vi "Build keyword and value string vector.vi"(1 "Keywords":string, 3 "Values":string) -> (15 "Keywords & Values in 128 Bytes vector":u8[](array[numeric]))   [LabVIEW 2022 SP3, in "RPC.lvclass"]
uses:
  RPC.lvclass
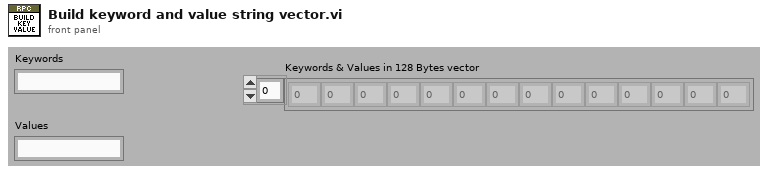
[diagram p1: front panel]
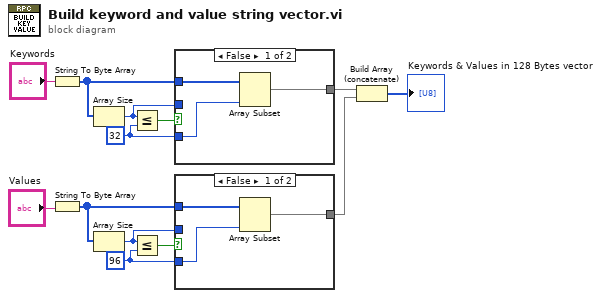
[diagram p0: block diagram]
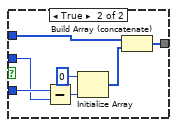
[diagram p2: hidden frame]
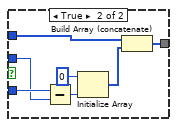
[diagram p3: hidden frame]
diagram:
  w7 = 96 ("y")
  w10 = 32 ("y")
  n1 = String To Byte Array(string="Keywords") -> (unsigned byte array=w11:u8[])
  n2 = String To Byte Array(string="Values") -> (unsigned byte array=w6:u8[])
  n3 = Array Size(array=w11) -> (size(s)=w9:i32)
  n4 = Array Size(array=w6) -> (size(s)=w8:i32)
  n5 = Less Or Equal?(x=w9, y=w10) -> (x <= y?=w12:bool)
  n6 = Less Or Equal?(x=w8, y=w7) -> (x <= y?=w5:bool)
  n7 = case shown="False" w12 {
    tunnel: w11 -> [w16 w19]
    tunnel: w10 -> [w15 w23]
    tunnel: [w14 w17] -> w3
    tunnel: w9 -> [_ w22]
    frame False {
      n8 = Array Subset(array=w16, length=w15) -> (w14:u8[])  [unwired: 1 in]
    }
    frame True {
      n9 = Subtract(x=w23, y=w22) -> (x-y=w21:i32)
      n10 = Initialize Array(u8 0 ("element"), w21) -> (w18:u8[])
      n11 = Build Array (concatenate)(w19, w18) -> (w17:u8[])
    }
  }
  n12 = case shown="False" w5 {
    tunnel: w6 -> [w26 w29]
    tunnel: w7 -> [w25 w33]
    tunnel: [w24 w27] -> w2
    tunnel: w8 -> [_ w32]
    frame False {
      n13 = Array Subset(array=w26, length=w25) -> (w24:u8[])  [unwired: 1 in]
    }
    frame True {
      n14 = Subtract(x=w33, y=w32) -> (x-y=w31:i32)
      n15 = Initialize Array(u8 0 ("element"), w31) -> (w28:u8[])
      n16 = Build Array (concatenate)(w29, w28) -> (w27:u8[])
    }
  }
  n17 = Build Array (concatenate)(w3, w2) -> (→"Keywords & Values in 128 Bytes vector":u8[])
